vi "GetNextWindow.vi"(8 "error in (no error)":errorcluster, 11 "hWnd (NULL)":T1) -> (0 "error out":errorcluster, 3 "hWnd":T1)   [LabVIEW 2011]
doc: "GetWindowText\nThe GetWindowText function copies the text of the specified window's title bar (if it has one) into a buffer. If the specified window is a control, the text of the control is copied. However, GetWindowText cannot retrieve the text of a control in another application.\n\nint GetWindowText(\n HWND hWnd, // handle to window or control with text\n LPTSTR lpString, // address of buffer for text\n int nMaxCount // maximum number of characters to copy\n);\n \nParameters\nhWnd \nHandle to the window or control containing the text. \nlpString \nPointer to the buffer that will receive the text. \nnMaxCount \nSpecifies the maximum number of characters to copy to the buffer, including the NULL character. If the text exceeds this limit, it is truncated. \nReturn Values\nIf the function succeeds, the return value is the length, in characters, of the copied string, not including the terminating null character. If the window has no title bar or text, if the title bar is empty, or if the window or control handle is invalid, the return value is zero. To get extended error information, callGetLastError. \n\nThis function cannot retrieve the text of an edit control in another application.\n\nRemarks\nIf the target window is owned by the current process, GetWindowText causes a WM_GETTEXT message to be sent to the specified window or control. If the target window is owned by another process and has a caption, GetWindowText retrieves the window caption text. If the window does not have a caption, the return value is a null string."
uses:
  hWnd.ctl
  user32.dll
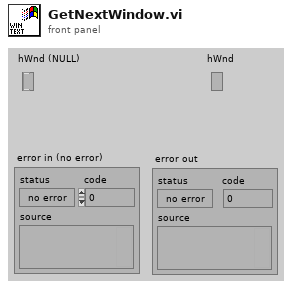
[diagram p1: front panel]
types:
  T1 = typedef "hWnd.ctl" = refnum<k1>
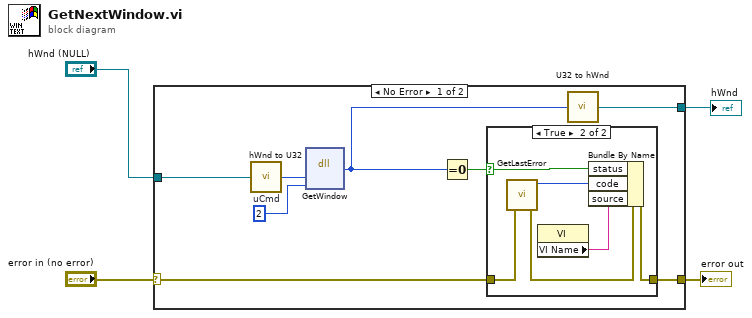
[diagram p0: block diagram]
diagram:
  n1 = case shown="No Error" "error in (no error)" {
    selector: "error in (no error)" -> [w11 w21]
    tunnel: "hWnd (NULL)" -> [w12 w20]
    tunnel: [w9 w21] -> w2
    tunnel: [w6 w20] -> w1
    frame No Error {
      w7 = u32 2  # uCmd
      n2 = call "hWnd to U32.vi"("hWnd"=w12) -> ("hWnd"=w8:u32)  [unwired: 4 out]
      n3 = dll-call lib="user32.dll" fn="GetWindow"("hWnd"=w8, "uCmd"=w7) -> ("return type"=w5:u32)  [unwired: 5 in, 2 out]
      n4 = Equal To 0?(x=w5) -> (x = 0?=w10:bool)
      n5 = case shown="True" w10 {
        selector: w10 -> [_ w18]
        tunnel: w11 -> [w13 w16]
        tunnel: [w13 w19] -> w9
        frame False {
        }
        frame True {
          n6 = call "GetLastError.vi"("error in (no error)"=w16) -> ("error out"=w15:errorcluster, "CODE"=w17:i32)  [unwired: 5 out]
          n7 = property class="VI"() -> ("VI Name"=w14:string)  [unwired: 2 in, 2 out]
          n8 = Bundle By Name(cluster=w15, "status"=w18, "code"=w17, "source"=w14) -> (w19:errorcluster)
        }
      }
      n9 = call "U32 to hWnd.vi"("hWnd"=w5) -> ("hWnd"=w6:T1)  [unwired: 4 out]
    }
    frame Error {
    }
  }
  "error out" <- w2
  "hWnd" <- w1
